vi "Module Cleanup.vi"(8 "error in (no error)":errorcluster, 11 "DAQmxDI in":refnum<class " DAQmxDI Port.lvclass">) -> (0 "error out":errorcluster, 3 "DAQmxDI out":refnum<class " DAQmxDI Port.lvclass">)   [LabVIEW 2020, in " DAQmxDI Port.lvclass"]
uses:
   DAQmxDI Port.lvclass
   DAQmxDI Port.lvclass/ DAQmxDI Port.ctl
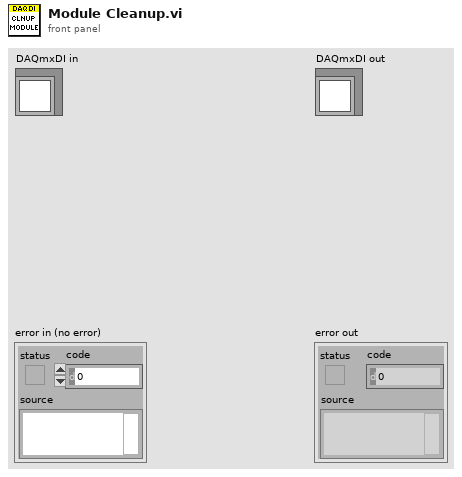
[diagram p1: front panel]
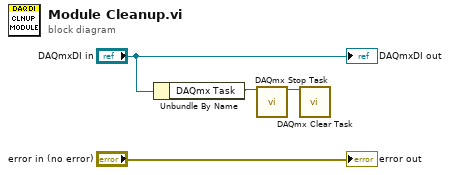
[diagram p0: block diagram]
diagram:
  n1 = Unbundle By Name("DAQmxDI in") -> ("DAQmx Task"=w3:refnum<k21>)
  n2 = call <vilib>:"DAQmx Stop Task.vi"("task/channels in"=w3) -> ("task out"=w2:refnum<k21>)  [unwired: 13 in, 1 out]
  n3 = call <vilib>:"DAQmx Clear Task.vi"("task in"=w2) -> ()  [unwired: 14 in, 1 out]
  "error out" <- "error in (no error)"
  "DAQmxDI out" <- "DAQmxDI in"
